vi "Synchio.Shutdown.vi"(8 "error in (no error)":errorcluster, 10 "AIAO Tasks":T1={"AI task"=["", ""], "AO Task"=[""]}, 11 "SynchIO in":refnum<class "SynchIO.lvclass">) -> (0 "error out":errorcluster, 3 "SynchIO out":refnum<class "SynchIO.lvclass">)   [LabVIEW 2016, in "SynchIO.lvclass"]
uses:
  SynchIO.lvclass
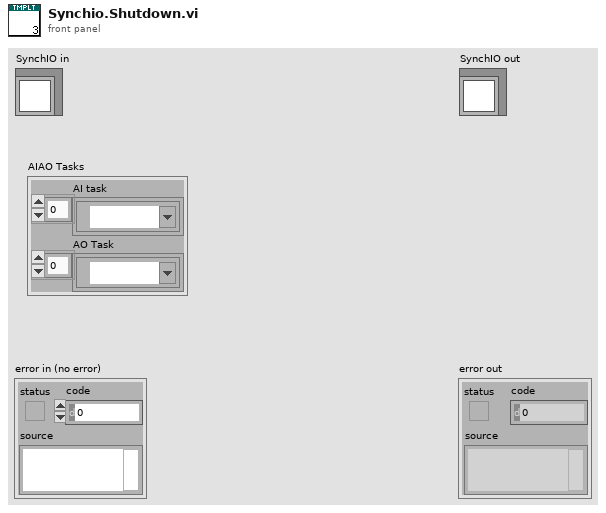
[diagram p1: front panel]
types:
  T1 = cluster{"AI task":refnum<k21>[], "AO Task":refnum<k21>[]}
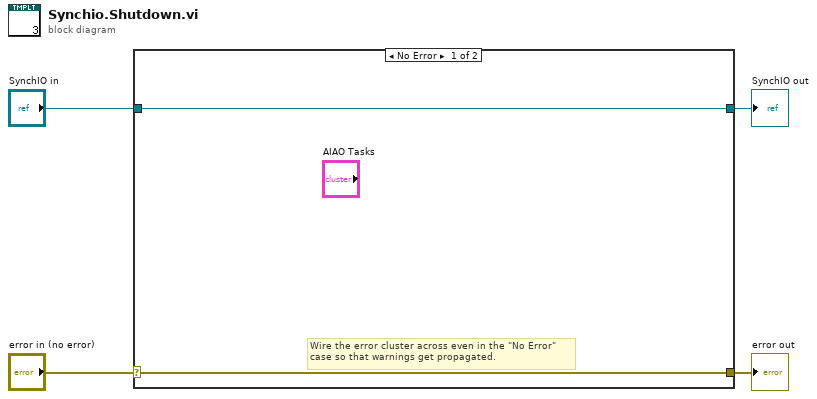
[diagram p0: block diagram]
diagram:
  n1 = case shown="No Error" "error in (no error)" {
    selector: "error in (no error)" -> [w5 w8]
    tunnel: [w5 w8] -> w3
    tunnel: [w6 w7] -> w1
    tunnel: "SynchIO in" -> [w6 w7]
    frame No Error {
      # "Wire the error cluster across even in the \"No Error\"\ncase so that warnings get propagated."
    }
    frame Error {
    }
  }
  "error out" <- w3
  "SynchIO out" <- w1
